vi "MotorTimeout(encoder).vi"() -> ()   [LabVIEW 2010]
uses:
  <vilib>/NXT/Subs/MotorXNode.DC Motor Type.ctl
  <vilib>/NXT/Subs/LVHSConnector.ctl
  <vilib>/NXT/NXTIO Xnodes/NXTIOXNode/NXTIO.xnode
  <vilib>/NXT/Subs/MotorXNode.2DCMotor.ctl
  <vilib>/NXT/NXTIO Xnodes/NXTIONodeSubVIs/TETRIX IO Motor Status.vi
  <vilib>/NXT/Dual Mode Library/Sound/PlayRedPianoFile.vi
  <vilib>/NXT/NXTIO Xnodes/NXTIONodeSubVIs/TETRIX IO Stop DC Motors.vi
panel:
  in  "Motors at Risk":T2
  in  "Encoder Motor":T2
  in  "Target Rate":i32
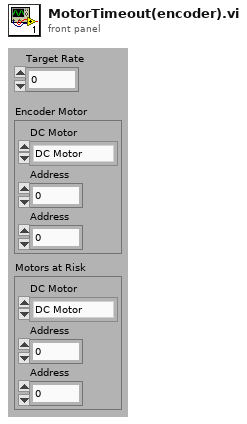
[diagram p1: front panel]
types:
  T1 = typedef "MotorXNode.DC Motor Type.ctl" = enum16{"DC Motor"}
  T2 = cluster{"DC Motor":T1, "Address":i16, "Address":i16}
  T3 = typedef "LVHSConnector.ctl" = cluster{"Hardware":string, "Flattened String":string}
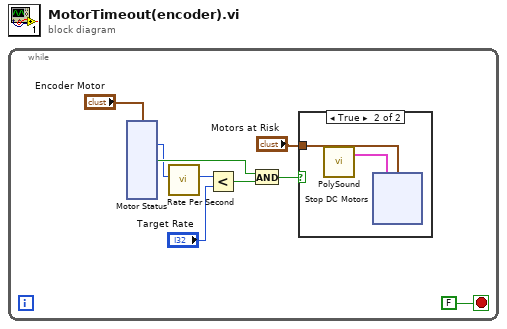
[diagram p0: block diagram]
diagram:
  n1 = while {
    stop <- FALSE stop-if-true
    n2 = xnode "Motor Status"("Motors"="Encoder Motor") -> ("Moving 1"=w7:bool, "Position 1"=w3:i32)  [unwired: 1 in, 3 out]
    n3 = call "Rate Per Second.vi"("Input Number"=w3) -> ("Rate Per Second"=w2:i32)  [unwired: 10 in]
    n4 = Less?(x=w2, y="Target Rate") -> (x < y?=w8:bool)
    n5 = And(x=w7, y=w8) -> (x .and. y?=w6:bool)
    n6 = case shown="True" w6 {
      tunnel: "Motors at Risk" -> [_ w10]
      frame False {
      }
      frame True {
        n7 = call-poly <vilib>:"PolySound.vi"() -> ("NXT"=w11:T3)  [unwired: 4 in]
        n8 = xnode "Stop DC Motors"("Motors"=w10, "NXT"=w11) -> ()  [unwired: 1 out]
      }
    }
  }
